vi "XimeaSetFramerate.vi"(8 "error in":errorcluster, 10 "ValueDBL":dbl=1.0 min=1.0 max=250.0 step=1.0, 11 "Session In":T1="cam5") -> (0 "error out":errorcluster)   [LabVIEW 2017, in "ImageAcquisitionLibrary.lvlib"]
uses:
  ImageAcquisitionProgram/ImageAcquisitionLibrary/ImageAcquisitionLibrary.lvlib
  <resource>/objmgr/imaqdx.rc
  <vilib>/vision/driver/NI_Vision_Acquisition_Software.lvlib
  <vilib>/userdefined/High Color/IMAQdx.ctl
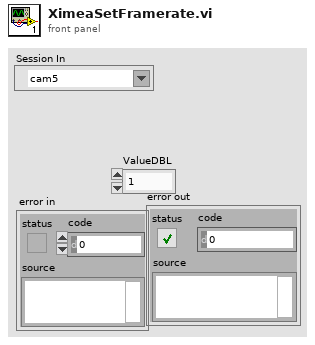
[diagram p1: front panel]
types:
  T1 = typedef "IMAQdx.ctl" = refnum<k21>
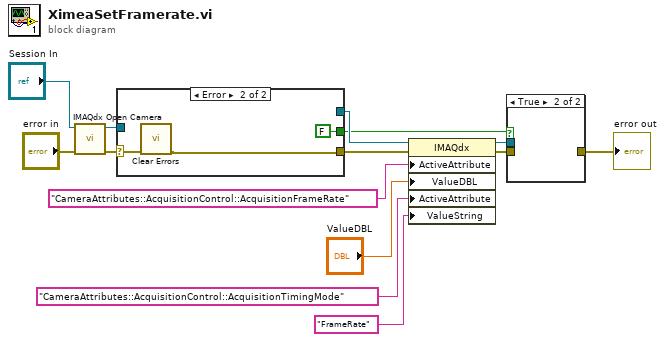
[diagram p0: block diagram]
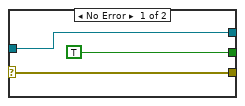
[diagram p3: hidden frame]
diagram:
  n1 = call <vilib>:"IMAQdx Open Camera.vi"("error in"="error in", "Session In"="Session In") -> ("error out"=w6:errorcluster, "Session Out"=w1:T1)  [unwired: 8 in]
  n2 = case shown="Error" w6 {
    selector: w6 -> [w16 w20]
    tunnel: [w16 w18] -> w5
    tunnel: [w17 _] -> w3
    tunnel: [TRUE FALSE] -> w2
    tunnel: w1 -> [w17 _]
    frame No Error {
    }
    frame Error {
      n3 = call <vilib>:"Clear Errors.vi"("error in (no error)"=w20) -> ("error out"=w18:errorcluster)  [unwired: 5 in, 1 out]
    }
  }
  n4 = property class="IMAQdx"(reference=w3, error in=w5, "ActiveAttribute"="CameraAttributes::AcquisitionControl::AcquisitionFrameRate", "ValueDBL"="ValueDBL", "ActiveAttribute"="CameraAttributes::AcquisitionControl::AcquisitionTimingMode", "ValueString"="FrameRate" ("ActiveAttribute")) -> (reference out=w9:T1, error out=w7:errorcluster)
  n5 = case shown="True" w2 {
    tunnel: w9 -> [_ _]
    tunnel: [w21 _] -> w8
    tunnel: w7 -> [w21 _]
    frame False {
    }
    frame True {
    }
  }
  "error out" <- w8
